vi "LV_receiver.vi"() -> ()   [LabVIEW 2019]
panel:
  out "data out":string
  in  "stop 2":bool
  out "port":u16
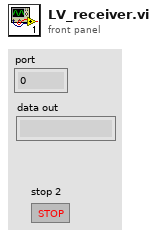
[diagram p1: front panel]
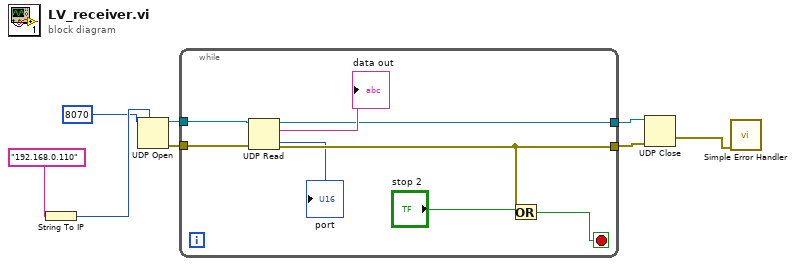
[diagram p0: block diagram]
diagram:
  n1 = String To IP(1:"192.168.0.110") -> (0:w5:u32)
  n2 = UDP Open(7:w5, 11:u16 8070 ("port")) -> (port=w3:refnum<k16>, 0:w2:errorcluster)  [unwired: 3 in, 1 out]
  n3 = while {
    tunnel: [w13] -> w8
    tunnel: [w12] -> w7
    tunnel: w3 -> [w11]
    tunnel: w2 -> [w10]
    stop <- w14 stop-if-true
    n4 = UDP Read(connection ID=w11, 8:w10) -> (data out=→"data out":string, error out=w13:errorcluster, 3:w12:refnum<k16>, 4:→"port":u16)  [unwired: 2 in, 1 out]
    n5 = Or(x=w13, y="stop 2") -> (x .or. y?=w14:bool)
  }
  n6 = UDP Close(connection ID=w7, 8:w8) -> (error out=w1:errorcluster)  [unwired: 1 out]
  n7 = call <vilib>:"Simple Error Handler.vi"("error in (no error)"=w1) -> ()  [unwired: 4 in, 5 out]
